vi "FT10_Connect FPGA_7854R Handler.vi"(8 "error in":errorcluster, 10 "Message Data":variant, 11 "Message Handling Cluster in":T1={"Fornax Connected?"=refnum, "Unitherm Connected?"=refnum, "M4X Connected?"=refnum, "Unitherm Connect/Disconnect"=refnum, "Fornax Connection"=refnum, "UNITHERM Connection"="", "M4X Connection"=0, "PXI-7854R FPGA Reference"=refnum, "PXI-7854R Connected?"=refnum, "Fornax Connect/Disconnect"=refnum, "7854 Connect/Disconnect"=refnum, "M4X Connect/Disconnect"=refnum, "Config Cluster"={"Unitherm Port"="COM4", "Simulate Values"=TRUE}, "Log Queue"=refnum, "Log Analysis Cluster"={"RMS"=0.0, "Envelope Frequency"=0.0, "Peak"=0.0, "Crest Factor"=0.0, "Duty Cyle %"=0.0, "P-P"=0.0, "Frequency"=0.0, "THD"=0.0, "Postive Peak"=0.0, "Negative Peak"=0.0, "Mag_H1"=0.0, "Phase_H1"=0.0, "Mag_H3"=0.0, "Phase_H3"=0.0, "Mag_H5"=0.0, "Phase_H5"=0.0}, "Log Waveform Cluster"={"t0"=timestamp(0 s since 1904-01-01), "dt"=1.0, "Y"=[]}, "Log Time"=timestamp(0 s since 1904-01-01), "Log Flag"=FALSE}) -> (0 "error out":errorcluster, 2 "PXI-7854R Connected?":bool, 3 "Message Handling Cluster out":T1={"Fornax Connected?"=refnum, "Unitherm Connected?"=refnum, "M4X Connected?"=refnum, "Unitherm Connect/Disconnect"=refnum, "Fornax Connection"=refnum, "UNITHERM Connection"="", "M4X Connection"=0, "PXI-7854R FPGA Reference"=refnum, "PXI-7854R Connected?"=refnum, "Fornax Connect/Disconnect"=refnum, "7854 Connect/Disconnect"=refnum, "M4X Connect/Disconnect"=refnum, "Config Cluster"={"Unitherm Port"="COM4", "Simulate Values"=TRUE}, "Log Queue"=refnum, "Log Analysis Cluster"={"RMS"=0.0, "Envelope Frequency"=0.0, "Peak"=0.0, "Crest Factor"=0.0, "Duty Cyle %"=0.0, "P-P"=0.0, "Frequency"=0.0, "THD"=0.0, "Postive Peak"=0.0, "Negative Peak"=0.0, "Mag_H1"=0.0, "Phase_H1"=0.0, "Mag_H3"=0.0, "Phase_H3"=0.0, "Mag_H5"=0.0, "Phase_H5"=0.0}, "Log Waveform Cluster"={"t0"=timestamp(0 s since 1904-01-01), "dt"=1.0, "Y"=[]}, "Log Time"=timestamp(0 s since 1904-01-01), "Log Flag"=FALSE})   [LabVIEW 2015]
uses:
  Controls/Control_Message Handling Cluster.ctl
  Controls/Control_M4X Connection.ctl
  Controls/Control_PXI-7854R FPGA Reference.ctl
  Controls/Control_Config Cluster.ctl
  Controls/Control_Config Unitherm Port.ctl
  Controls/Control_Config Simulate Values.ctl
  Controls/Control_Log Queue.ctl
  Controls/Control_Log Cluster.ctl
  Controls/Control_Log Time.ctl
  Controls/Control_Log Waveform Cluster.ctl
  Controls/Control_Log Analysis Cluster.ctl
  Controls/Control_Log Flag.ctl
  Controls/Control_PXI-7854R Connect Disconnect Cluster.ctl
  Controls/Control_PXI-7854R Resource.ctl
  Controls/Control_PXI-7854R 75kHz Bool.ctl
  Controls/Control_PXI-7854R uSec Off Numeric.ctl
  Controls/Control_PXI-7854R uSec On Numeric.ctl
  Controls/Control_PXI-7854R Connect Disconnect Bool.ctl
  <vilib>/FPGAPlugInAG/Dynamic/niLvFpga_Close_Dynamic.vi
  <vilib>/FPGAPlugInAG/PXI-7854R/niLvFpga_Open_PXI-7854R.vi
  <vilib>/rvi/interface/common/dynamic/niFpgaDynamicAddResources.vi
  <vilib>/Utility/error.llb/Error Cluster From Error Code.vi
  <vilib>/rvi/errors/niLvFpgaAdjustHostInterfaceError.vi
  <vilib>/rvi/interface/nirviCloseFPGA/nirviCloseFPGA.xnode
  <vilib>/rvi/interface/nirviOpenFPGA/nirviOpenFPGA.xnode
  FPGA Bitfiles/5_21_2024_FT10_FPGA_7854R_Main BitFile.lvbitx
  <vilib>/rvi/interface/nirviReadWriteControl/nirviReadWriteControl.xnode
  NiFpgaLv.dll
  <vilib>/rvi/interface/Simulation/niFpgaSimulationCallBeginRW.vi
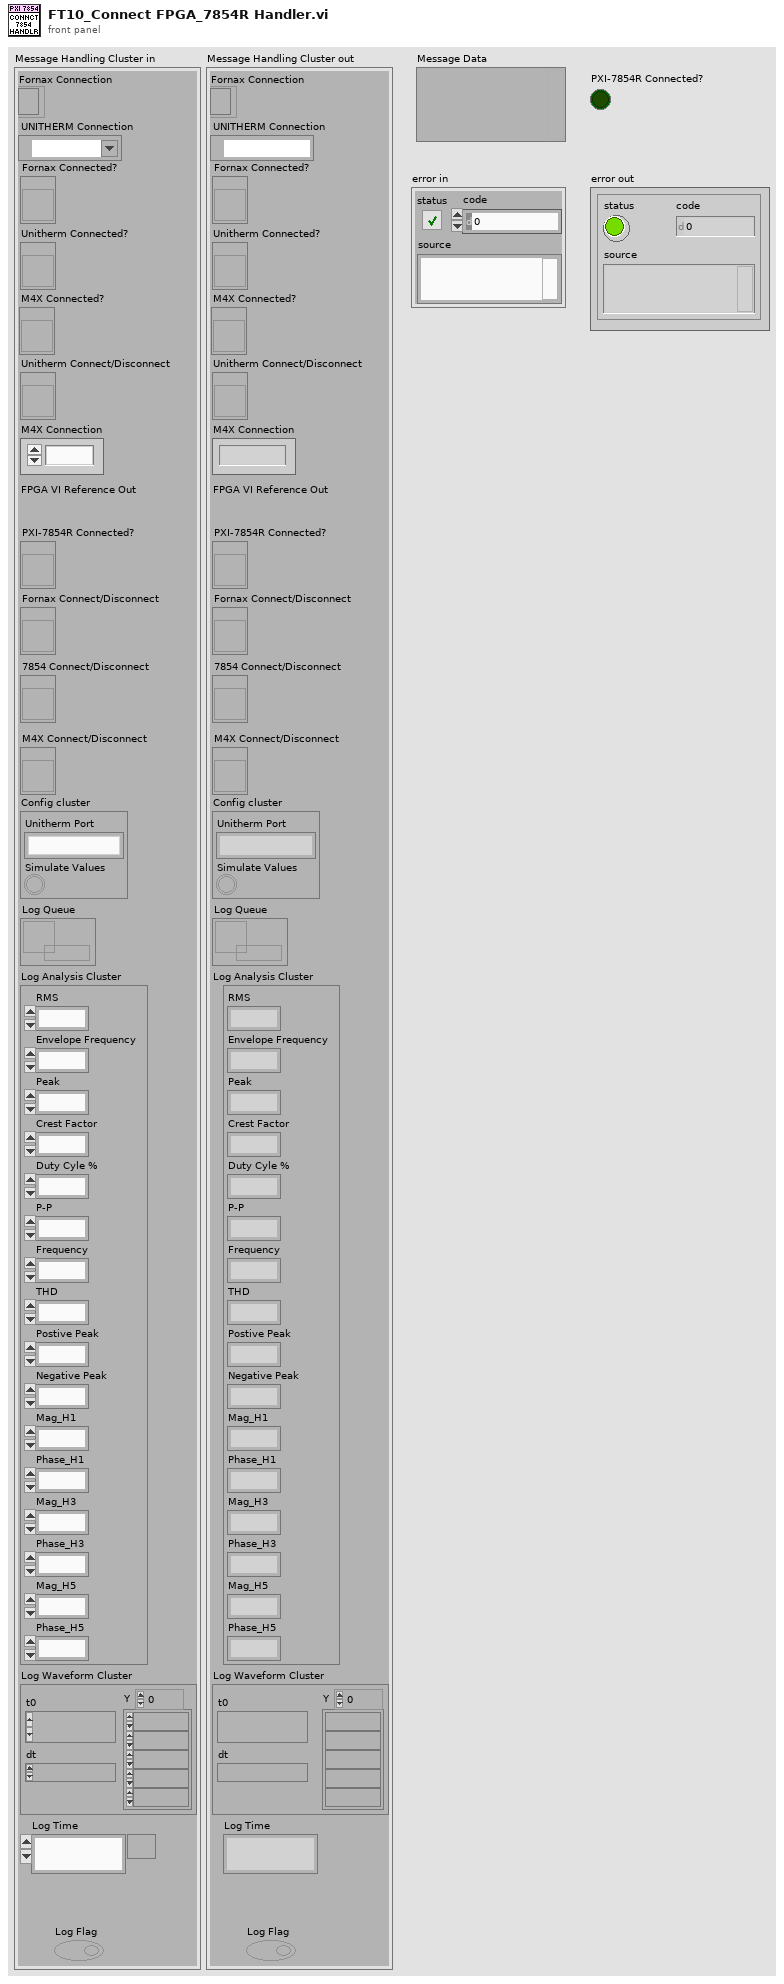
[diagram p1: front panel]
types:
  T1 = typedef "Control_Message Handling Cluster.ctl" = cluster{"Fornax Connected?":refnum<vi>, "Unitherm Connected?":refnum<vi>, "M4X Connected?":refnum<vi>, "Unitherm Connect/Disconnect":refnum<vi>, "Fornax Connection":refnum<k5>, "UNITHERM Connection":refnum<visa-resource-name>, "M4X Connection":T2, "PXI-7854R FPGA Reference":T3, "PXI-7854R Connected?":refnum<vi>, "Fornax Connect/Disconnect":refnum<vi>, "7854 Connect/Disconnect":refnum<vi>, "M4X Connect/Disconnect":refnum<vi>, "Config Cluster":T4, "Log Queue":T7, "Log Analysis Cluster":T8, "Log Waveform Cluster":T9, "Log Time":T10, "Log Flag":T11}
  T2 = typedef "Control_M4X Connection.ctl" = u32
  T3 = typedef "Control_PXI-7854R FPGA Reference.ctl" = refnum<k20>
  T4 = typedef "Control_Config Cluster.ctl" = cluster{"Unitherm Port":T5, "Simulate Values":T6}
  T5 = typedef "Control_Config Unitherm Port.ctl" = string
  T6 = typedef "Control_Config Simulate Values.ctl" = bool
  T7 = typedef "Control_Log Queue.ctl" = refnum<queue>
  T8 = typedef "Control_Log Analysis Cluster.ctl" = cluster{"RMS":dbl, "Envelope Frequency":dbl, "Peak":dbl, "Crest Factor":dbl, "Duty Cyle %":dbl, "P-P":dbl, "Frequency":dbl, "THD":dbl, "Postive Peak":dbl, "Negative Peak":dbl, "Mag_H1":dbl, "Phase_H1":dbl, "Mag_H3":dbl, "Phase_H3":dbl, "Mag_H5":dbl, "Phase_H5":dbl}
  T9 = typedef "Control_Log Waveform Cluster.ctl" = waveform(dbl)
  T10 = typedef "Control_Log Time.ctl" = timestamp
  T11 = typedef "Control_Log Flag.ctl" = bool
  T12 = typedef "Control_PXI-7854R Connect Disconnect Cluster.ctl" = cluster{"PXI-7854R Resource":T13, "75kHz":T14, "uSec Off":T15, "uSec On":T16, "7854 Connect/Disconnect":T17}
  T13 = typedef "Control_PXI-7854R Resource.ctl" = tag
  T14 = typedef "Control_PXI-7854R 75kHz Bool.ctl" = bool
  T15 = typedef "Control_PXI-7854R uSec Off Numeric.ctl" = u16
  T16 = typedef "Control_PXI-7854R uSec On Numeric.ctl" = u16
  T17 = typedef "Control_PXI-7854R Connect Disconnect Bool.ctl" = bool
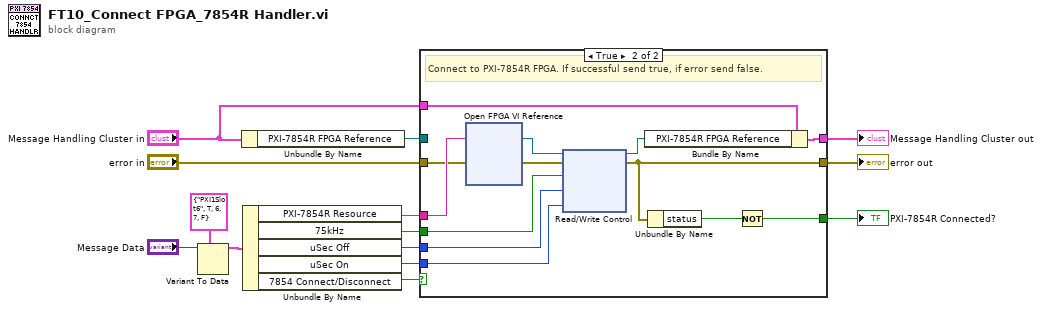
[diagram p0: block diagram]
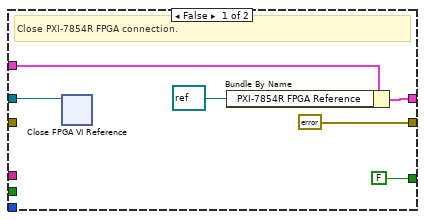
[diagram p2: hidden frame]
diagram:
  n1 = Variant To Data(type=T12 {"PXI-7854R Resource"="PXI1Slot6", "75kHz"=TRUE, "uSec Off"=6, "uSec On"=7, "7854 Connect/Disconnect"=FALSE}, Variant="Message Data") -> (data=w7:T12)  [unwired: 1 in, 1 out]
  n2 = Unbundle By Name("Message Handling Cluster in") -> ("PXI-7854R FPGA Reference"=w4:T3)
  n3 = Unbundle By Name(w7) -> ("PXI-7854R Resource"=w12:T13, "75kHz"=w8:T14, "uSec Off"=w9:T15, "uSec On"=w10:T16, "7854 Connect/Disconnect"=w11:T17)
  n4 = case shown="True" w11 {
    tunnel: w8 -> [_ w33]
    tunnel: w9 -> [_ w32]
    tunnel: w10 -> [_ w31]
    tunnel: w4 -> [w19 _]
    tunnel: [errorcluster {"status"=FALSE, "code"=0, "source"=""} ("error out") w23] -> w14
    tunnel: w12 -> [_ w29]
    tunnel: "error in" -> [_ w27]
    tunnel: "Message Handling Cluster in" -> [w18 w26]
    tunnel: [w17 w24] -> w2
    tunnel: [FALSE w21] -> w1
    frame False {
      # "Close PXI-7854R FPGA connection."
      n5 = xnode "Close FPGA VI Reference"("FPGA VI Reference In"=w19) -> ()  [unwired: 1 in, 1 out]
      n6 = Bundle By Name(cluster=w18, "PXI-7854R FPGA Reference"=refnum<k20> refnum ("FPGA VI Reference Out")) -> (w17:T1)
    }
    frame True {
      # "Connect to PXI-7854R FPGA. If successful send true, if error send false."
      n7 = xnode "Open FPGA VI Reference"("error in"=w27, "resource name"=w29) -> ("FPGA VI Reference Out"=w30:refnum<k20>, "error out"=w28:errorcluster)
      n8 = xnode "Read/Write Control"("FPGA VI Reference In"=w30, "error in"=w28, "75kHz"=w33, "uSec Off"=w32, "uSec On"=w31) -> ("FPGA VI Reference Out"=w25:refnum<k20>, "error out"=w23:errorcluster)
      n9 = Bundle By Name(cluster=w26, "PXI-7854R FPGA Reference"=w25) -> (w24:T1)
      n10 = Unbundle By Name(w23) -> ("status"=w22:bool)
      n11 = Not(x=w22) -> (.not. x?=w21:bool)
    }
  }
  "error out" <- w14
  "Message Handling Cluster out" <- w2
  "PXI-7854R Connected?" <- w1
